vi "Set Collect Aggregates Property.vi"(8 "error in (no error)":errorcluster, 10 "collect aggregates":bool, 11 "tags in":refnum<class "NI Skyline Tag.lvclass">[](array[class])) -> (0 "error out":errorcluster)   [LabVIEW 2020, in "FlexLoggerTagHelpers.lvlib"]
doc: "Indexes through the array of data, converting each element to a string based on it's data type."
uses:
  FlexLoggerTagHelpers.lvlib
  <vilib>/Skyline/Tag/Wrapper/Wrapper_class/NI Skyline Tag.lvclass
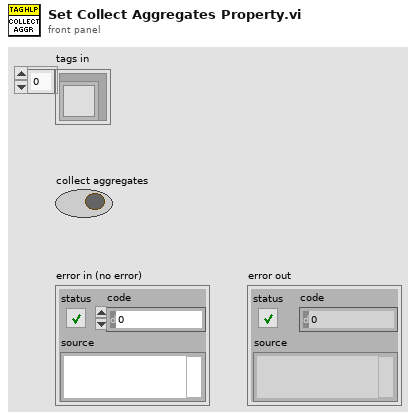
[diagram p1: front panel]
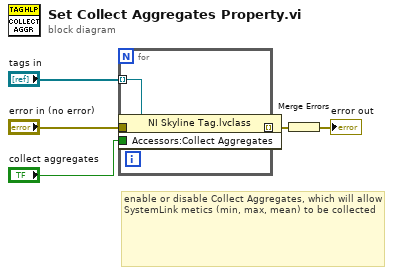
[diagram p0: block diagram]
diagram:
  # "enable or disable Collect Aggregates, which will allow SystemLink metics (min, max, mean) to be collected"
  n1 = for {
    tunnel: "tags in" -> [w8] mode=indexing
    tunnel: "collect aggregates" -> [w9]
    tunnel: "error in (no error)" -> [w7]
    tunnel: [w6] -> w3 mode=indexing
    n2 = property on="Property Node" class="NI Skyline Tag.lvclass"(reference=w8, error in=w7, "Accessors:Collect Aggregates"=w9) -> (error out=w6:errorcluster)  [unwired: 1 out]
  }
  n3 = Merge Errors(w3) -> (→"error out":errorcluster)
